vi "Linear_Array_NumSteps.vi"() -> ()   [LabVIEW 2022 SP3]
panel:
  out "Array":dbl[](array[numeric])
  in  "Number of Steps":dbl
  in  "Stop":dbl
  in  "Start":dbl
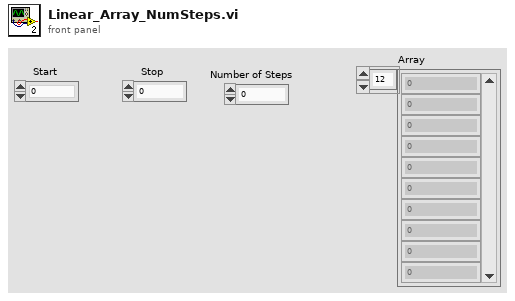
[diagram p1: front panel]
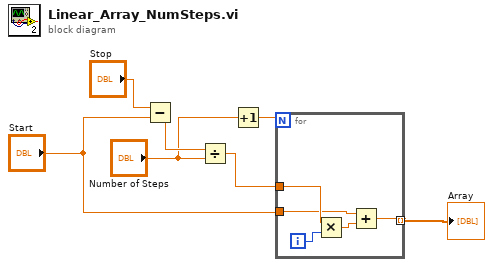
[diagram p0: block diagram]
diagram:
  n1 = Subtract(x="Stop", y="Start") -> (x-y=w6:dbl)
  n2 = Divide(x=w6, y="Number of Steps") -> (x/y=w3:dbl)
  n3 = Increment(x="Number of Steps") -> (x+1=w5:dbl)
  n4 = for {
    N: w5 -> [_]
    tunnel: [w8] -> w4 mode=indexing
    tunnel: w3 -> [w11]
    tunnel: "Start" -> [w9]
    i -> [w12]
    n5 = Multiply(x=w11, y=w12) -> (x*y=w10:dbl)
    n6 = Add(x=w9, y=w10) -> (x+y=w8:dbl)
  }
  "Array" <- w4
